vi "Task Init.vi"(8 "error in (no error)":errorcluster, 11 "ChartGuiTask in":refnum<class "ChartGuiTask.lvclass">) -> (0 "error out":errorcluster, 3 "ChartGuiTask out":refnum<class "ChartGuiTask.lvclass">)   [LabVIEW 2020, in "VolatusDemo.lvlib" / "ChartGuiTask.lvclass"]
uses:
  ChartGuiTask.lvclass
  ChartGuiTask.lvclass/ChartGuiTask.ctl
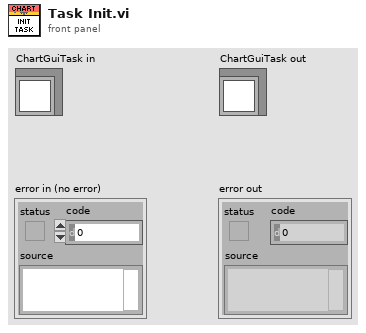
[diagram p1: front panel]
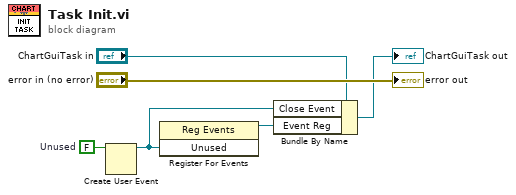
[diagram p0: block diagram]
diagram:
  w5 = FALSE  # Unused
  n1 = Create User Event(user event datatype=w5) -> (user event=w3:refnum<user-event>)  [unwired: 1 in, 1 out]
  n2 = register-events(w3) -> (reference out=w4:refnum<event-registration>)  [unwired: 2 in, 1 out]
  n3 = Bundle By Name(cluster="ChartGuiTask in", "Close Event"=w3, "Event Reg"=w4) -> (→"ChartGuiTask out":refnum<class "ChartGuiTask.lvclass">)
  "error out" <- "error in (no error)"
